vi "Merge_Raw_DF_metadata.vi"(4 "New Values In":string[](array[string]), 5 "New Chs In":string[](array[string]), 6 "Orig Values In":string[][](array[string]), 7 "Orig Chs In":string[](array[string])) -> (0 "Channel Values Out":string[][](array[string]), 1 "Ch names Out":string[](array[string]), 3 "Original values":string[](array[string]))   [LabVIEW 2010]
panel:
  out "Case":string
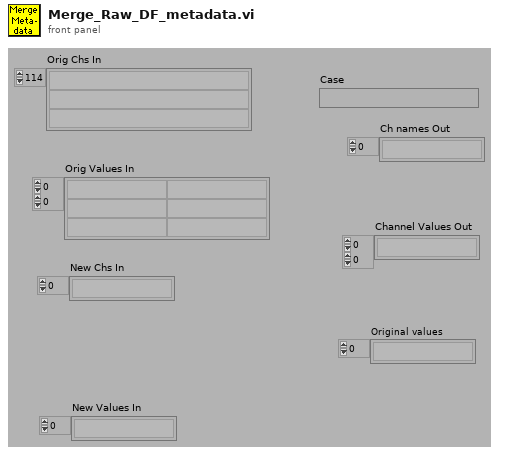
[diagram p1: front panel]
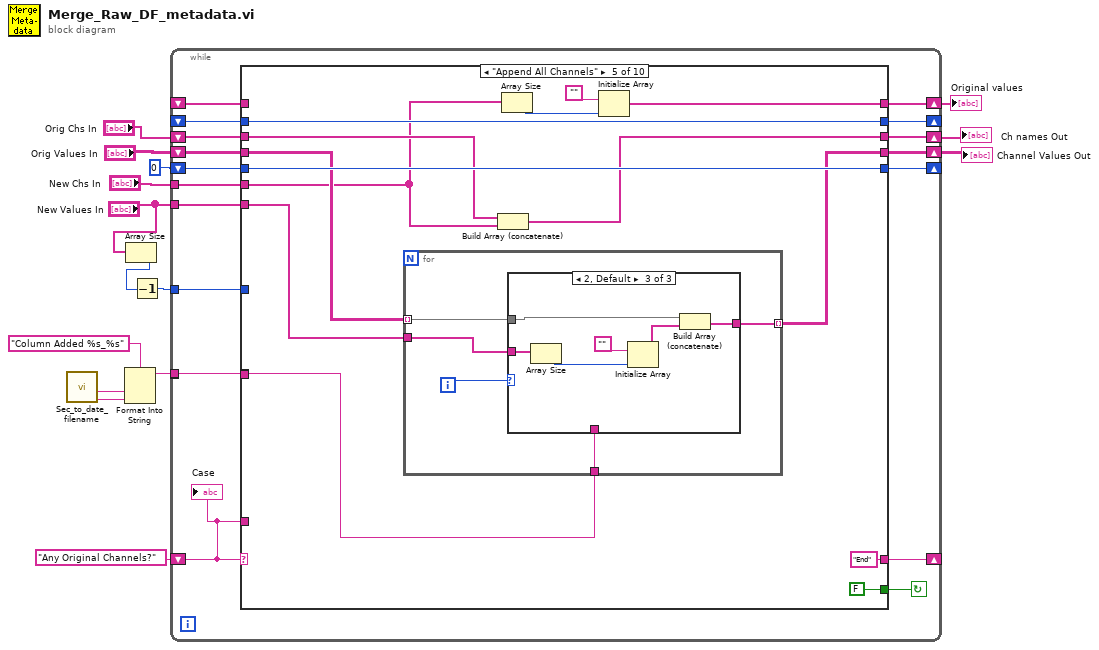
[diagram p0: block diagram]
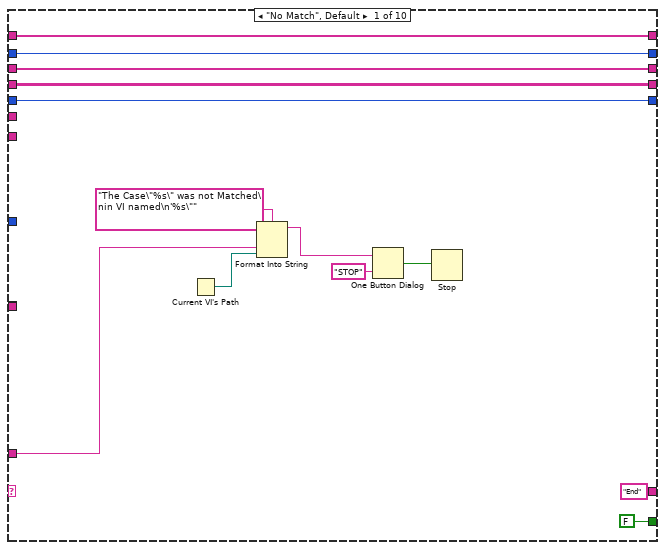
[diagram p2: hidden frame]
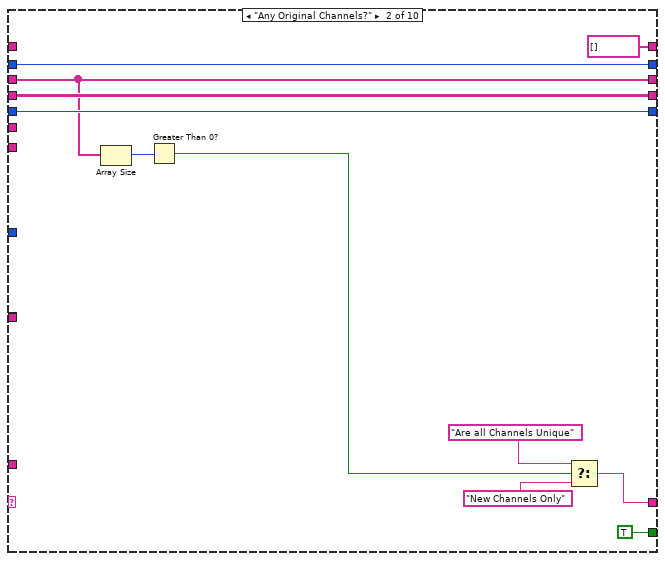
[diagram p3: hidden frame]
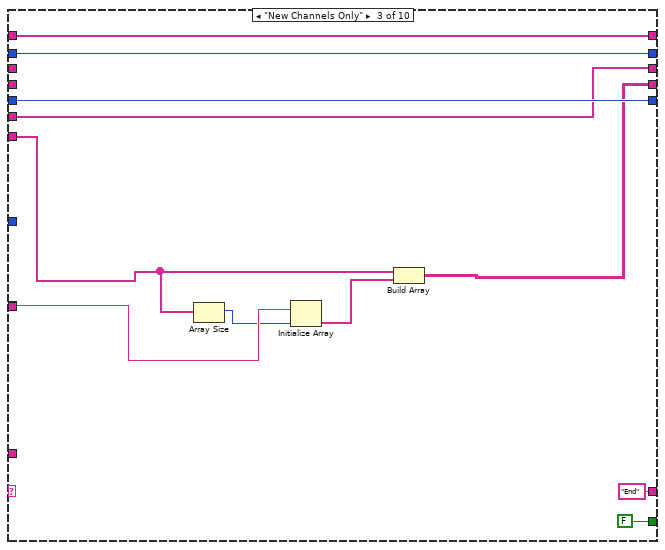
[diagram p4: hidden frame]
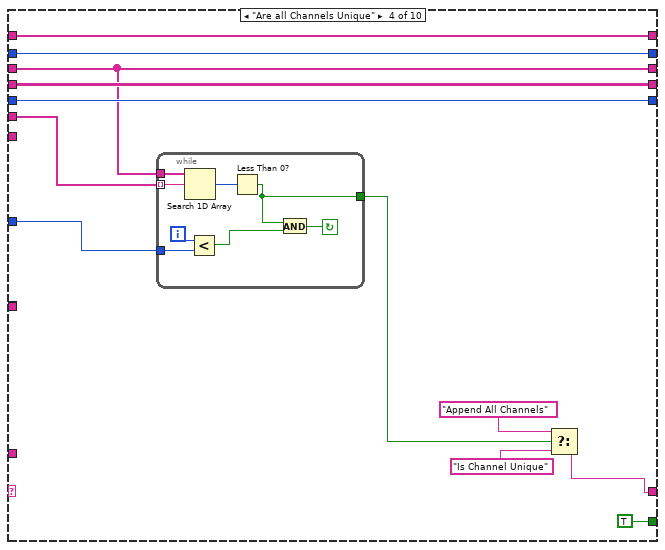
[diagram p5: hidden frame]
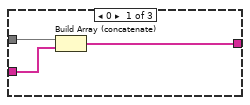
[diagram p6: hidden frame]
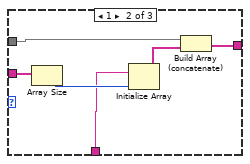
[diagram p7: hidden frame]
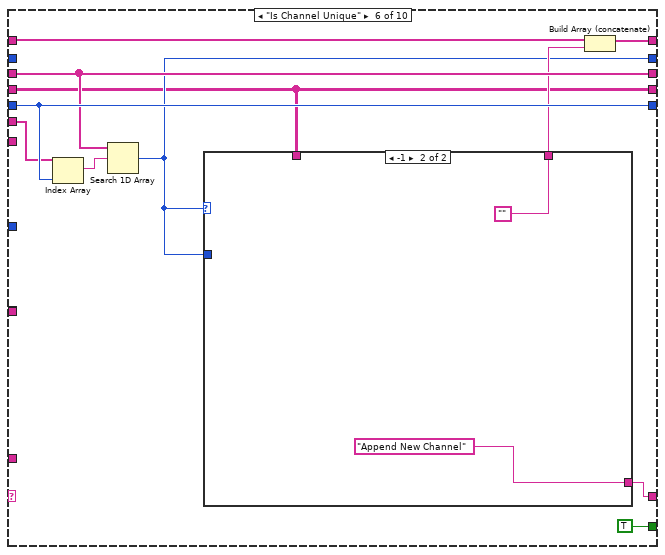
[diagram p8: hidden frame]
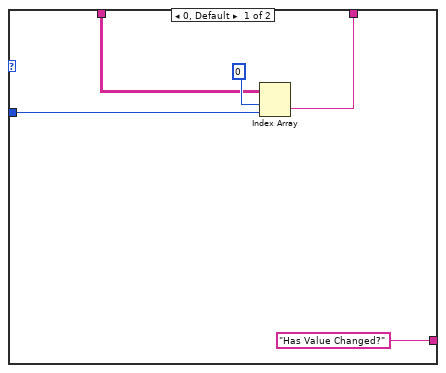
[diagram p9: hidden frame]
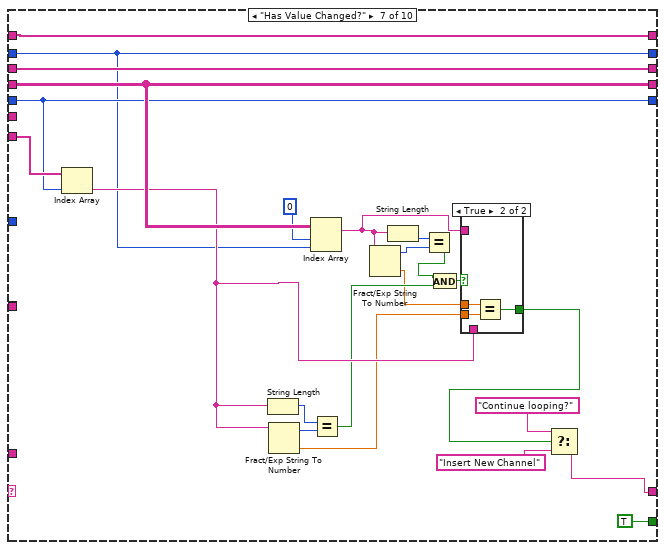
[diagram p10: hidden frame]
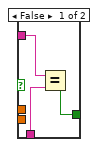
[diagram p11: hidden frame]
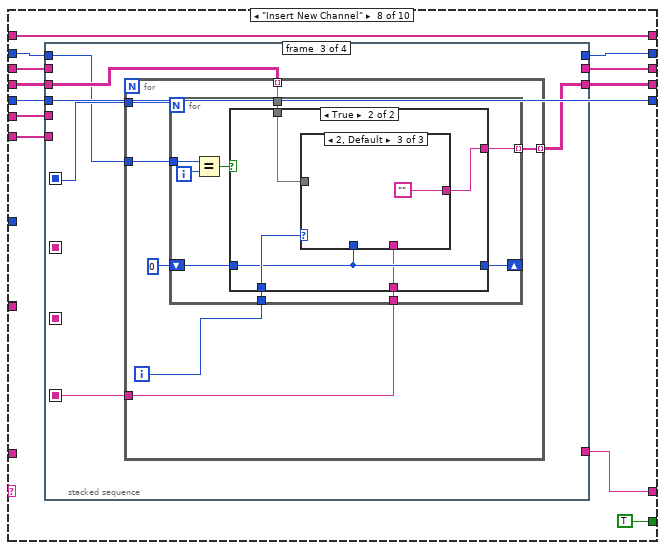
[diagram p12: hidden frame]
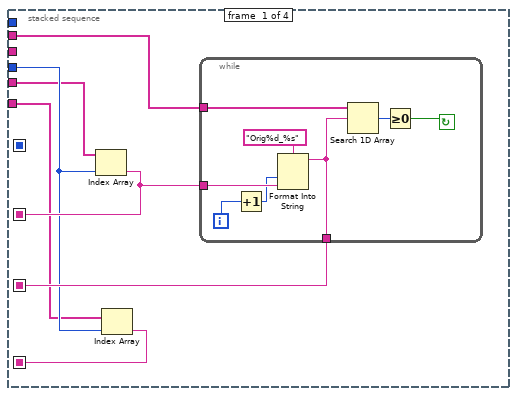
[diagram p13: hidden frame]
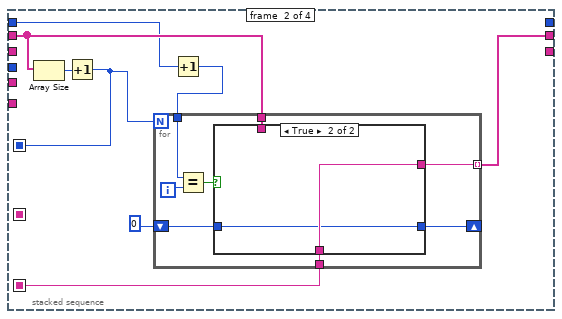
[diagram p14: hidden frame]
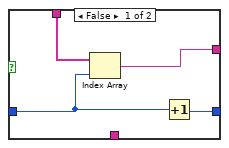
[diagram p15: hidden frame]
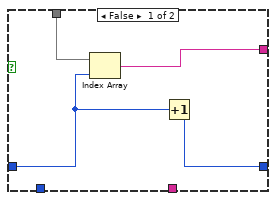
[diagram p16: hidden frame]
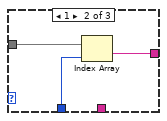
[diagram p18: hidden frame]
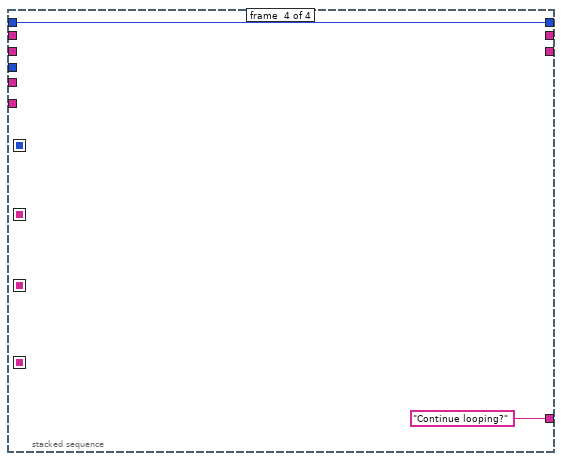
[diagram p19: hidden frame]
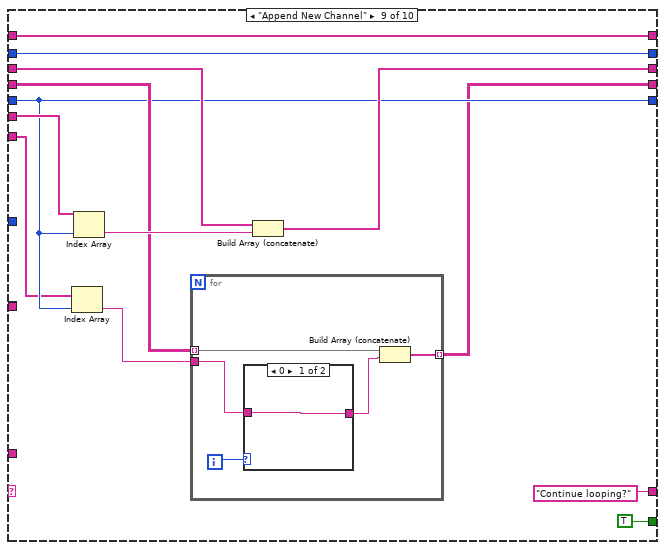
[diagram p20: hidden frame]
diagram:
  n1 = call "Sec_to_date_filename.vi"() -> ("Day"=w4:string, "Time"=w1:string)  [unwired: 1 in, 2 out]
  n2 = Format Into String(format string="Column Added %s_%s" ("Format String"), w4, w1) -> (resulting string=w5:string)  [unwired: 2 in, 1 out]
  n3 = Array Size(array="New Values In") -> (size(s)=w11:i32)
  n4 = Decrement(x=w11) -> (x-1=w10:i32)
  n5 = while {
    tunnel: w5 -> [w18]
    tunnel: w5 -> [w19]
    shift-left: _ -> [w21]
    shift-right: [w20] -> _
    tunnel: "New Values In" -> [w22]
    tunnel: "New Chs In" -> [w23]
    tunnel: w10 -> [w24]
    shift-left: 0 -> [w25]
    shift-right: [w26] -> _
    shift-left: "Orig Values In" -> [w28]
    shift-right: [w27] -> w13
    shift-left: "Orig Chs In" -> [w29]
    shift-right: [w30] -> w14
    shift-left: "Any Original Channels?" -> [w32]
    shift-right: [w31] -> _
    shift-right: [w16] -> w2
    shift-left: _ -> [w17]
    stop <- w33 continue-if-true
    n6 = case shown="\"Append All Channels\"" w32 {
      tunnel: [FALSE ("Results File?") TRUE ("Results File?") FALSE ("Results File?") TRUE ("Results File?") FALSE ("Results File?") TRUE ("Results File?") TRUE ("Results File?") TRUE ("Results File?") TRUE ("Results File?") w281] -> w33
      tunnel: w32 -> [w41 _ _ _ _ _ _ _ _ _]
      tunnel: w23 -> [_ _ w63 w73 w90 w128 _ w178 w267 _]
      tunnel: w22 -> [_ _ w62 _ w96 _ w160 w177 w261 _]
      tunnel: ["End" w52 "End" ("f") w79 "End" ("f") w132 w161 w173 "Continue looping?" "Is Channel Unique"] -> w31
      tunnel: [w38 w50 w63 w74 w98 w129 w163 w174 w264 w283] -> w30
      tunnel: w29 -> [w38 w50 _ w74 w99 w129 w163 w180 w265 w283]
      tunnel: w28 -> [w37 w56 _ w78 w97 w123 w159 w175 w263 w284]
      tunnel: [w37 w56 w64 w78 w95 w123 w159 w176 w259 w284] -> w27
      tunnel: [w36 w55 w67 w77 w101 w131 w151 w179 w262 w278] -> w26
      tunnel: w25 -> [w36 w55 w67 w77 w101 w131 w151 w179 w262 w279]
      tunnel: w24 -> [_ _ _ w72 _ _ _ _ _ w282]
      tunnel: w21 -> [w35 w54 w66 w70 w94 _ w150 w172 w257 w277]
      tunnel: [w35 w54 w66 w70 w94 w124 w150 w171 w257 w277] -> w20
      tunnel: w19 -> [_ _ w61 _ w93 _ _ _ _ _]
      tunnel: w18 -> [_ _ _ _ _ _ _ _ _ _]
      tunnel: w17 -> [w34 _ w58 w69 _ w126 w141 w170 w256 w276]
      tunnel: [w34 string[] [] w58 w69 w89 w125 w141 w170 w256 w276] -> w16
      frame "No Match", Default {
        n7 = Current VI's Path() -> (path=w42:path)
        n8 = Format Into String(format string="The Case\"%s\" was not Matched\nin VI named\n'%s\"" ("Format String"), w41, w42) -> (resulting string=w45:string)  [unwired: 2 in, 1 out]
        n9 = One Button Dialog(message=w45, button name ("OK")="STOP") -> (true=w43:bool)
        n10 = Stop(stop? (T)=w43) -> ()
      }
      frame "Any Original Channels?" {
        n11 = Array Size(array=w50) -> (size(s)=w49:i32)
        n12 = Greater Than 0?(x=w49) -> (x > 0?=w48:bool)
        n13 = Select(t="Are all Channels Unique", s=w48, f="New Channels Only") -> (s? t:f=w52:string)
      }
      frame "New Channels Only" {
        n14 = Array Size(array=w62) -> (size(s)=w60:i32)
        n15 = Initialize Array(w61, w60) -> (w59:string[])
        n16 = Build Array(w62, w59) -> (w64:string[][])
      }
      frame "Are all Channels Unique" {
        n17 = while {
          tunnel: [w81] -> w71
          tunnel: w72 -> [w84]
          tunnel: w73 -> [w87] mode=indexing
          tunnel: w74 -> [w88]
          i -> [w85]
          stop <- w82 continue-if-true
          n18 = Search 1D Array(1D array=w88, element=w87) -> (index of element=w86:i32)  [unwired: 1 in]
          n19 = Less?(x=w85, y=w84) -> (x < y?=w83:bool)
          n20 = Less Than 0?(x=w86) -> (x < 0?=w81:bool)
          n21 = And(x=w81, y=w83) -> (x .and. y?=w82:bool)
        }
        n22 = Select(t="Append All Channels" ("f"), s=w71, f="Is Channel Unique") -> (s? t:f=w79:string)
      }
      frame "Append All Channels" {
        n23 = for {
          tunnel: w97 -> [w107] mode=indexing
          tunnel: w96 -> [w106]
          tunnel: [w105] -> w95 mode=indexing
          tunnel: w93 -> [w104]
          i -> [w103]
          n24 = case shown="2, Default" w103 {
            tunnel: w107 -> [w110 w112 w119]
            tunnel: w106 -> [w109 w116 w122]
            tunnel: [w108 w111 w118] -> w105
            tunnel: w104 -> [_ w114 _]
            frame 0 {
              n25 = Build Array (concatenate)(w110, w109) -> (w108:string[])
            }
            frame 1 {
              n26 = Array Size(array=w116) -> (size(s)=w115:i32)
              n27 = Initialize Array(w114, w115) -> (w113:string[])
              n28 = Build Array (concatenate)(w112, w113) -> (w111:string[])
            }
            frame 2, Default {
              n29 = Array Size(array=w122) -> (size(s)=w121:i32)
              n30 = Initialize Array("", w121) -> (w120:string[])
              n31 = Build Array (concatenate)(w119, w120) -> (w118:string[])
            }
          }
        }
        n32 = Build Array (concatenate)(w99, w90) -> (w98:string[])
        n33 = Array Size(array=w90) -> (size(s)=w91:i32)
        n34 = Initialize Array("", w91) -> (w89:string[])
      }
      frame "Is Channel Unique" {
        n35 = Index Array(array=w128, index=w131) -> (element=w130:string)
        n36 = Search 1D Array(1D array=w129, element=w130) -> (index of element=w124:i32)  [unwired: 1 in]
        n37 = case shown="-1" w124 {
          tunnel: ["Has Value Changed?" ("f") "Append New Channel"] -> w132
          tunnel: [w136 ""] -> w127
          tunnel: w124 -> [w137 _]
          tunnel: w123 -> [w135 _]
          frame 0, Default {
            n38 = Index Array(array=w135, index (row)=0, index (col)=w137) -> (element=w136:string)
          }
          frame -1 {
          }
        }
        n39 = Build Array (concatenate)(w126, w127) -> (w125:string[])
      }
      frame "Has Value Changed?" {
        n40 = Index Array(array=w160, index=w151) -> (element=w154:string)
        n41 = String Length(string=w154) -> (length=w156:i32)
        n42 = Fract/Exp String To Number(string=w154) -> (offset past number=w155:i32, number=w152:dbl)  [unwired: 3 in]
        n43 = Index Array(array=w159, index (row)=0, index (col)=w150) -> (element=w144:string)
        n44 = Equal?(x=w156, y=w155) -> (x = y?=w153:bool)
        n45 = Fract/Exp String To Number(string=w144) -> (offset past number=w148:i32, number=w145:dbl)  [unwired: 3 in]
        n46 = String Length(string=w144) -> (length=w149:i32)
        n47 = Equal?(x=w149, y=w148) -> (x = y?=w147:bool)
        n48 = And(x=w147, y=w153) -> (x .and. y?=w146:bool)
        n49 = case shown="True" w146 {
          tunnel: w145 -> [_ w169]
          tunnel: w152 -> [_ w168]
          tunnel: [w164 w167] -> w142
          tunnel: w144 -> [w166 _]
          tunnel: w154 -> [w165 _]
          frame False {
            n50 = Equal?(x=w166, y=w165) -> (x = y?=w164:bool)
          }
          frame True {
            n51 = Equal?(x=w169, y=w168) -> (x = y?=w167:bool)
          }
        }
        n52 = Select(t="Continue looping?", s=w142, f="Insert New Channel") -> (s? t:f=w161:string)
      }
      frame "Insert New Channel" {
        n53 = stacked-sequence {
          seq-local: [w187 _ _ _] -> [_ _ _ _]
          seq-local: [w186 _ _ _] -> [_ w199 _ _]
          seq-local: [w183 _ _ _] -> [_ _ w222 _]
          seq-local: [_ w201 _ _] -> [_ _ w220 _]
          tunnel: w180 -> [w188 w202 _ _]
          tunnel: w179 -> [w185 _ _ _]
          tunnel: w178 -> [w182 _ _ _]
          tunnel: w177 -> [w184 _ _ _]
          tunnel: [_ _ w223 _] -> w176
          tunnel: w175 -> [_ _ w221 _]
          tunnel: [_ w200 _ _] -> w174
          tunnel: [_ _ _ "Continue looping?"] -> w173
          tunnel: w172 -> [_ w198 w219 w254]
          tunnel: [_ _ _ w254] -> w171
          frame #0 {
            n54 = Index Array(array=w182, index=w185) -> (element=w187:string)
            n55 = Index Array(array=w184, index=w185) -> (element=w183:string)
            n56 = while {
              tunnel: [w189] -> w186
              tunnel: w187 -> [w195]
              tunnel: w188 -> [w196]
              i -> [w191]
              stop <- w192 continue-if-true
              n57 = Increment(x=w191) -> (x+1=w190:i32)
              n58 = Format Into String(format string="Orig%d_%s" ("Format String"), w190, w195) -> (resulting string=w189:string)  [unwired: 2 in, 1 out]
              n59 = Search 1D Array(1D array=w196, element=w189) -> (index of element=w193:i32)  [unwired: 1 in]
              n60 = Greater Or Equal To 0?(x=w193) -> (x >= 0?=w192:bool)
            }
          }
          frame #1 {
            n61 = Array Size(array=w202) -> (size(s)=w204:i32)
            n62 = Increment(x=w204) -> (x+1=w201:i32)
            n63 = Increment(x=w198) -> (x+1=w197:i32)
            n64 = for {
              N: w201 -> [_]
              shift-right: [w207] -> _
              shift-left: 0 -> [w208]
              tunnel: [w210] -> w200 mode=indexing
              tunnel: w199 -> [w209]
              tunnel: w202 -> [w206]
              tunnel: w197 -> [w205]
              i -> [w212]
              n65 = Equal?(x=w205, y=w212) -> (x = y?=w211:bool)
              n66 = case shown="True" w211 {
                tunnel: [w215 w218] -> w210
                tunnel: w209 -> [_ w218]
                tunnel: w206 -> [w216 _]
                tunnel: w208 -> [w214 w217]
                tunnel: [w213 w217] -> w207
                frame False {
                  n67 = Index Array(array=w216, index=w214) -> (element=w215:string)
                  n68 = Increment(x=w214) -> (x+1=w213:i32)
                }
                frame True {
                }
              }
            }
          }
          frame #2 {
            n69 = for {
              tunnel: w220 -> [w229]
              tunnel: w219 -> [w228]
              tunnel: [w227] -> w223 mode=indexing
              tunnel: w222 -> [w225]
              tunnel: w221 -> [w226] mode=indexing
              i -> [w224]
              n70 = for {
                N: w229 -> [_]
                shift-right: [w233] -> _
                shift-left: 0 -> [w234]
                tunnel: w228 -> [w238]
                tunnel: [w236] -> w227 mode=indexing
                tunnel: w226 -> [w235]
                tunnel: w224 -> [w232]
                tunnel: w225 -> [w231]
                i -> [w239]
                n71 = Equal?(x=w238, y=w239) -> (x = y?=w237:bool)
                n72 = case shown="True" w237 {
                  tunnel: [w242 w245] -> w236
                  tunnel: w235 -> [w243 w246]
                  tunnel: w234 -> [w241 w247]
                  tunnel: [w240 w247] -> w233
                  tunnel: w232 -> [_ w248]
                  tunnel: w231 -> [_ w244]
                  frame False {
                    n73 = Index Array(array=w243, index=w241) -> (element=w242:string)
                    n74 = Increment(x=w241) -> (x+1=w240:i32)
                  }
                  frame True {
                    n75 = case shown="2, Default" w248 {
                      tunnel: w247 -> [_ w252 _]
                      tunnel: w246 -> [_ w251 _]
                      tunnel: [w249 w250 ""] -> w245
                      tunnel: w244 -> [w249 _ _]
                      frame 0 {
                      }
                      frame 1 {
                        n76 = Index Array(array=w251, index=w252) -> (element=w250:string)
                      }
                      frame 2, Default {
                      }
                    }
                  }
                }
              }
            }
          }
          frame #3 {
          }
        }
      }
      frame "Append New Channel" {
        n77 = Index Array(array=w261, index=w262) -> (element=w260:string)
        n78 = Index Array(array=w267, index=w262) -> (element=w266:string)
        n79 = for {
          tunnel: w263 -> [w273] mode=indexing
          tunnel: w260 -> [w269]
          tunnel: [w272] -> w259 mode=indexing
          i -> [w271]
          n80 = case shown="0" w271 {
            tunnel: [w274 ""] -> w270
            tunnel: w269 -> [w274 _]
            frame 0 {
            }
            frame 1, Default {
            }
          }
          n81 = Build Array (concatenate)(w273, w270) -> (w272:string[])
        }
        n82 = Build Array (concatenate)(w265, w266) -> (w264:string[])
      }
      frame "Continue looping?" {
        n83 = Less?(x=w279, y=w282) -> (x < y?=w281:bool)
        n84 = Increment(x=w279) -> (x+1=w278:i32)
      }
    }
    "Case" <- w32
  }
  "Channel Values Out" <- w13
  "Ch names Out" <- w14
  "Original values" <- w2
